vi "CRYProject Popup Menu.vi"(8 "Tree Reference In":refnum<vi>, 9 "Coords In":T1, 10 "This VI":refnum<vi>, 11 "Menu Ref In":refnum<k9>) -> (0 "Tree Reference Out":refnum<vi>, 3 "Menu Ref Out":refnum<k9>)   [LabVIEW 2013]
uses:
  <vilib>/Utility/miscctls.llb/LVPoint32TypeDef.ctl
  CRYMainGlobal.vi
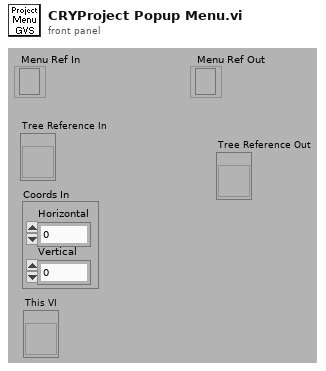
[diagram p1: front panel]
types:
  T1 = typedef "LVPoint32TypeDef.ctl" = cluster{"Horizontal":i32, "Vertical":i32}
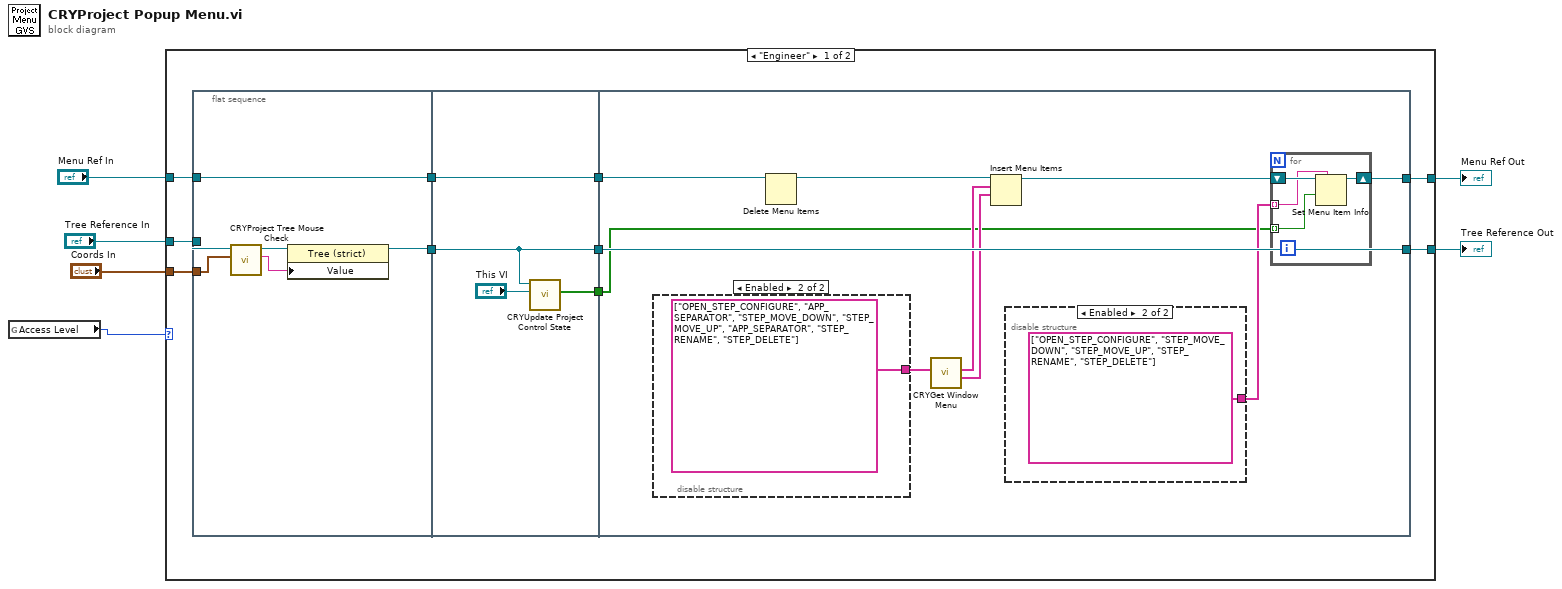
[diagram p0: block diagram]
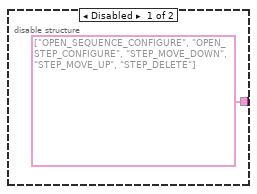
[diagram p2: hidden frame]
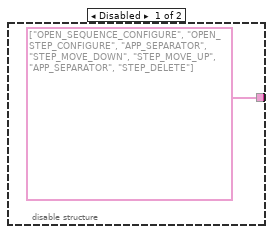
[diagram p3: hidden frame]
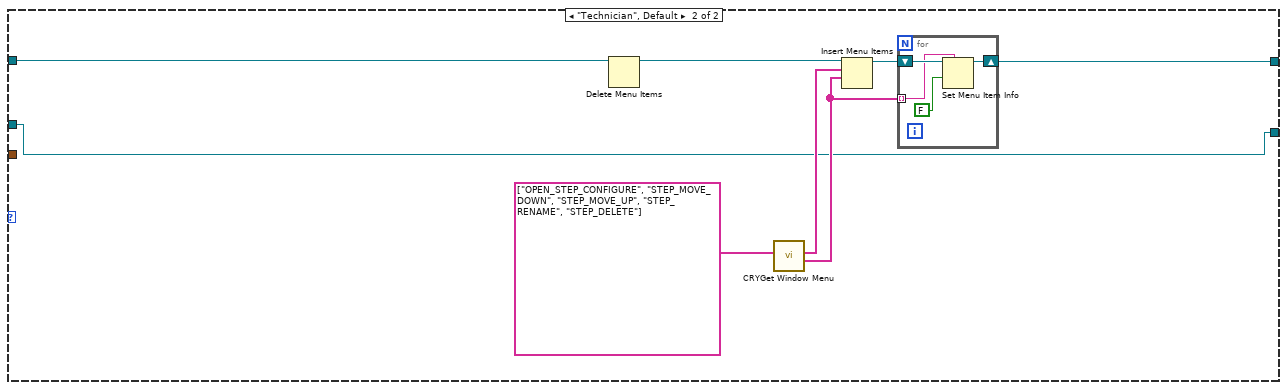
[diagram p4: hidden frame]
diagram:
  n1 = global read "CRYMainGlobal.vi" "Access Level"() -> (w1:enum16{"Engineer", "Technician", "Operator"})
  n2 = case shown="\"Engineer\"" w1 {
    tunnel: "Tree Reference In" -> [w11 w45]
    tunnel: "Coords In" -> [w10 _]
    tunnel: [w9 w51] -> w4
    tunnel: "Menu Ref In" -> [w8 w52]
    tunnel: [w7 w45] -> w2
    frame "Engineer" {
      n3 = flat-sequence {
        tunnel: w11 -> [w17]
        tunnel: w10 -> [w21]
        tunnel: [w22] -> w16
        tunnel: w8 -> [w22]
        tunnel: [w19] -> w15
        tunnel: w16 -> [w26]
        tunnel: [w26] -> w14
        tunnel: w15 -> [w24]
        tunnel: [w24] -> w13
        tunnel: [w23] -> w12
        tunnel: [w32] -> w9
        tunnel: w14 -> [w35]
        tunnel: [w34] -> w7
        tunnel: w13 -> [w34]
        tunnel: w12 -> [w27]
        frame #0 {
          n4 = call "CRYProject Tree Mouse Check.vi"("Coords In"=w21, "Tree Reference In"=w17) -> ("Clicked String Out"=w18:string, "Tree Reference Out"=w20:refnum<vi>)  [unwired: 8 in]
          n5 = property class="Tree (strict)"(reference=w20, "Value"=w18) -> (reference out=w19:refnum<vi>)  [unwired: 1 in, 1 out]
        }
        frame #1 {
          n6 = call "CRYUpdate Project Control State.vi"("VI Ref"="This VI", "RefTree In"=w24) -> ("State FlgArray"=w23:bool[])  [unwired: 8 in, 1 out]
        }
        frame #2 {
          n7 = disable-structure shown="Enabled" {
            disable-tunnel: [string[] ["OPEN_SEQUENCE_CONFIGURE", "OPEN_STEP_CONFIGURE", "APP_SEPARATOR", "STEP_MOVE_DOWN", "STEP_MOVE_UP", "APP_SEPARATOR", "STEP_DELETE"] ("item tags") string[] ["OPEN_STEP_CONFIGURE", "APP_SEPARATOR", "STEP_MOVE_DOWN", "STEP_MOVE_UP", "APP_SEPARATOR", "STEP_RENAME", "STEP_DELETE"] ("item tags")] -> w30
            frame Disabled {
            }
            frame Enabled {
            }
          }
          n8 = Delete Menu Items(9:w35) -> (3:w36:refnum<k9>)  [unwired: 2 in, 2 out]
          n9 = call "CRYGet Window Menu.vi"("Tags"=w30) -> ("Tags_Out"=w28:string[], "Names_Out"=w29:string[])  [unwired: 8 in, 1 out]
          n10 = Insert Menu Items(7:w28, 8:w29, 9:w36) -> (3:w33:refnum<k9>)  [unwired: 1 in, 4 out]
          n11 = disable-structure shown="Enabled" {
            disable-tunnel: [string[] ["OPEN_SEQUENCE_CONFIGURE", "OPEN_STEP_CONFIGURE", "STEP_MOVE_DOWN", "STEP_MOVE_UP", "STEP_DELETE"] ("item tags") string[] ["OPEN_STEP_CONFIGURE", "STEP_MOVE_DOWN", "STEP_MOVE_UP", "STEP_RENAME", "STEP_DELETE"] ("item tags")] -> w31
            frame Disabled {
            }
            frame Enabled {
            }
          }
          n12 = for {
            tunnel: w31 -> [w42] mode=indexing
            shift-right: [w43] -> w32
            shift-left: w33 -> [w44]
            tunnel: w27 -> [w41] mode=indexing
            n13 = Set Menu Item Info(7:w42, 9:w41, 11:w44) -> (3:w43:refnum<k9>)  [unwired: 3 in, 2 out]
          }
        }
      }
    }
    frame "Technician", Default {
      n14 = Delete Menu Items(9:w52) -> (3:w50:refnum<k9>)  [unwired: 2 in, 2 out]
      n15 = call "CRYGet Window Menu.vi"("Tags"=string[] ["OPEN_STEP_CONFIGURE", "STEP_MOVE_DOWN", "STEP_MOVE_UP", "STEP_RENAME", "STEP_DELETE"] ("item tags")) -> ("Tags_Out"=w46:string[], "Names_Out"=w47:string[])  [unwired: 8 in, 1 out]
      n16 = Insert Menu Items(7:w46, 8:w47, 9:w50) -> (3:w49:refnum<k9>)  [unwired: 1 in, 4 out]
      n17 = for {
        tunnel: w46 -> [w54] mode=indexing
        shift-right: [w55] -> w51
        shift-left: w49 -> [w56]
        n18 = Set Menu Item Info(7:w54, 9:FALSE ("enabled"), 11:w56) -> (3:w55:refnum<k9>)  [unwired: 3 in, 2 out]
      }
    }
  }
  "Menu Ref Out" <- w4
  "Tree Reference Out" <- w2
